vi "mxwScript_API_XMLTemplateName_AddFirstDropPosition.vi"(8 "error in (no error)":errorcluster, 10 "distance":i32=10 min=0, 11 "absolutePath":string) -> (0 "error out":errorcluster, 3 "encoded absolutePath":string)   [LabVIEW 2020]
doc: "Sets the drop parameters to drop this template below all code on the current root block diagram."
uses:
  codeGenAPISupport.llb/cgAPI_mxwScript_DrpTmplt_TemplateRefType.ctl
  codeGenAPISupport.llb/cgAPI_mxwScript_DrpTmplt_ReferencePosition.ctl
  codeGenAPISupport.llb/cgAPI_mxwScript_DrpTmplt_TargetRefType.ctl
  codeGenAPISupport.llb/cgAPI_mxwScript_DrpTmplt_SimpleDirection.ctl
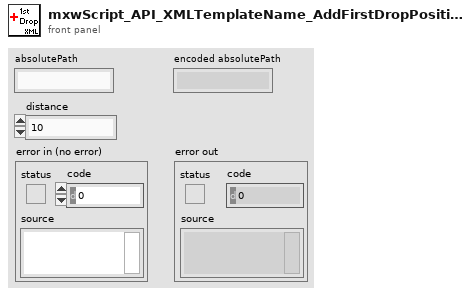
[diagram p1: front panel]
types:
  T1 = typedef "cgAPI_mxwScript_DrpTmplt_SimpleDirection.ctl" = enum16{"Right", "Left", "Below", "Above"}
  T2 = typedef "cgAPI_mxwScript_DrpTmplt_ReferencePosition.ctl" = enum16{"TopLeft", "Top", "TopRight", "Left", "Middle", "Right", "BottomLeft", "Bottom", "BottomRight"}
  T3 = typedef "cgAPI_mxwScript_DrpTmplt_TargetRefType.ctl" = enum16{"RelativeToTemplate", "RelativeToTerminal", "AbsoluteOnRoot", "AbsoluteOnTarget", "RelativeToExistOnRoot"}
  T4 = typedef "cgAPI_mxwScript_DrpTmplt_TemplateRefType.ctl" = enum16{"InputAverage", "Absolute", "Terminal"}
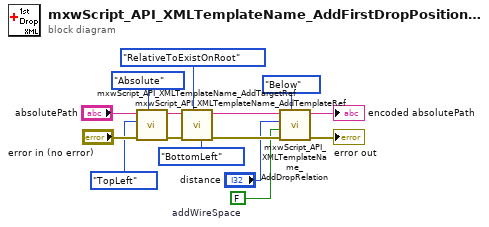
[diagram p0: block diagram]
diagram:
  w3 = FALSE  # addWireSpace
  n1 = call "mxwScript_API_XMLTemplateName_AddTemplateRef.vi"("templateRefType"=cgAPI_mxwScript_DrpTmplt_TemplateRefType."Absolute", "error in (no error)"="error in (no error)", "referencePosition"=cgAPI_mxwScript_DrpTmplt_ReferencePosition."TopLeft", "absolutePath"="absolutePath") -> ("error out"=w11:errorcluster, "encoded absolutePath"=w10:string)  [unwired: 1 in, 5 out]
  n2 = call "mxwScript_API_XMLTemplateName_AddTargetRef.vi"("relativeToExistData"=cgAPI_mxwScript_DrpTmplt_ReferencePosition."BottomLeft", "targetRefType"=cgAPI_mxwScript_DrpTmplt_TargetRefType."RelativeToExistOnRoot", "error in (no error)"=w11, "absolutePath"=w10) -> ("error out"=w7:errorcluster, "encoded absolutePath"=w6:string)  [unwired: 3 in, 3 out]
  n3 = call "mxwScript_API_XMLTemplateName_AddDropRelation.vi"("direction"=cgAPI_mxwScript_DrpTmplt_SimpleDirection."Below", "error in (no error)"=w7, "addWireSpace"=w3, "distance"="distance", "absolutePath"=w6) -> ("error out"=→"error out":errorcluster, "encoded absolutePath"=→"encoded absolutePath":string)  [unwired: 5 out]
